vi "Get Vector - stdout.vi"(6 "no transpose\nfor reading":bool, 8 "error in (no error)":errorcluster, 9 "octave vector sizes":i32[](array[numeric]), 10 "variable name":string, 11 "GOLPI ref. in":T1={"pipe handle"={"lv_proc.dll file path"=path "", "process instance handle"=[]}, "fast read timeout [ms]"=500, "fast read settle time [ms]"=10, "fast read to multiple [ms]"=1, "max elements per input line"=100, "slow read timeout [ms]"=5000}) -> (0 "error out":errorcluster, 2 "vector":string[](array[string]), 3 "GOLPI ref. out":T1={"pipe handle"={"lv_proc.dll file path"=path "", "process instance handle"=[]}, "fast read timeout [ms]"=500, "fast read settle time [ms]"=10, "fast read to multiple [ms]"=1, "max elements per input line"=100, "slow read timeout [ms]"=5000}, 4 "value transposed?":bool)   [LabVIEW 2013, in "GOLPI library.lvlib"]
doc: "Reads vector variable from GNU Octave. Returns output as array of strings. Internaly converts row vector to column for simpler parsing of long vectors. It means complex vectors are conjugated and strings are incorrectly parsed. If 'no transpose for reading' is set true, function reads row vectors as rows."
uses:
  GOLPI library.lvlib
  Type Definitions/GOLPI reference Type Def.ctl
  LV Process.lvlibp/Pipe Handle.ctl
  Type Definitions/Custom Error Codes Enum Type Def.vi
  LV Process.lvlibp
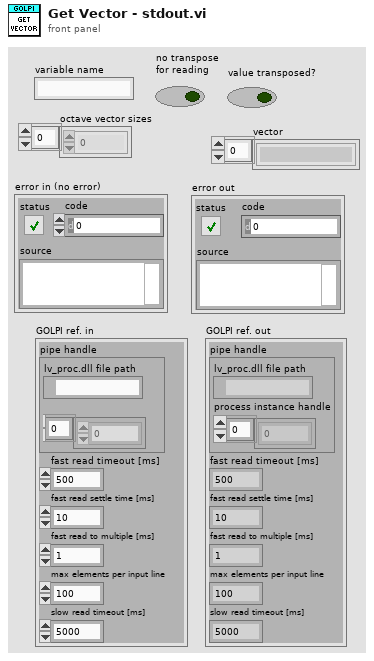
[diagram p1: front panel]
types:
  T1 = typedef "GOLPI library.lvlib/GOLPI reference Type Def.ctl" = cluster{"pipe handle":T2, "fast read timeout [ms]":u32, "fast read settle time [ms]":u32, "fast read to multiple [ms]":u32, "max elements per input line":u32, "slow read timeout [ms]":u32}
  T2 = typedef "LV Process.lvlibp/Pipe Handle.ctl" = cluster{"lv_proc.dll file path":path, "process instance handle":u32[]}
  T3 = typedef "GOLPI library.lvlib/Custom Error Codes Enum Type Def.vi" = enum16{"no error", "00 working directory PAR1 missing", "01 octave binary PAR1 missing", "02 octave report error PAR1", "03 empty output last cmd PAR1", "04 missing temporary file PAR1", "05 pwd PAR 1 not exist", "10 var PAR1 not string", "11 var PAR1 not num, scal, ~compl", "12 var PAR1 not num, scal, compl", "13 var PAR1 not num, vect, ~compl", "14 var PAR1 not num, vect, compl", "15 var PAR1 not num, mat, ~compl", "16 var PAR1 not num, mat, ~compl", "30 WARNING read timeout", "99 not finished"}
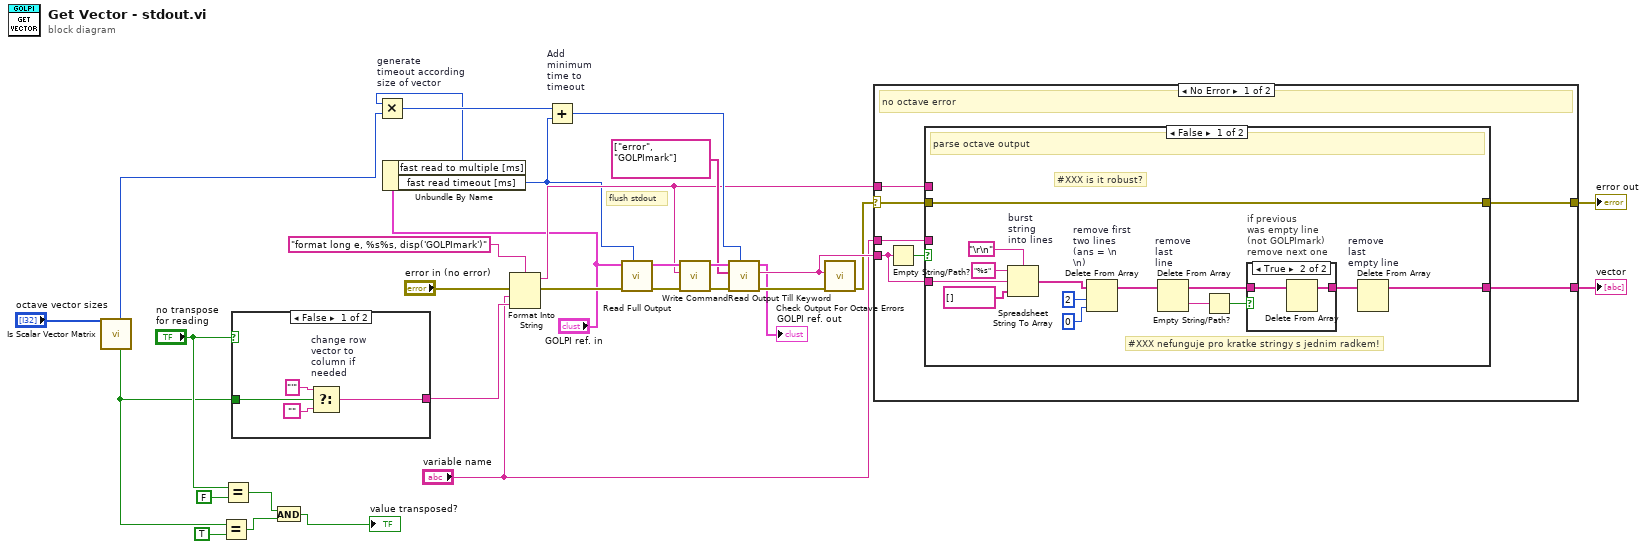
[diagram p0: block diagram]
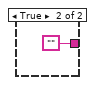
[diagram p2: hidden frame]
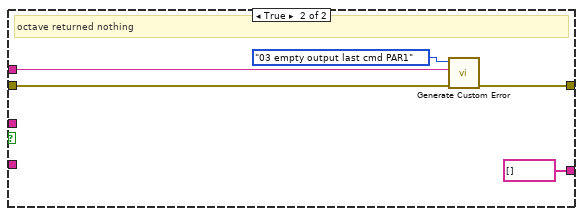
[diagram p4: hidden frame]
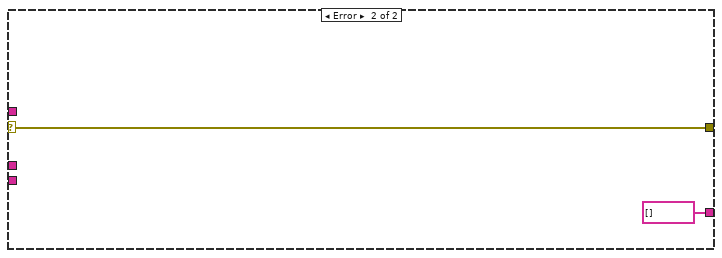
[diagram p5: hidden frame]
diagram:
  # "flush stdout"
  n1 = call "Is Scalar Vector Matrix.vi"("octave sizes"="octave vector sizes") -> ("row vector?"=w4:bool, "vector length"=w12:i32)  [unwired: 5 in, 4 out]
  n2 = Equal?(x=w4, y=TRUE) -> (x = y?=w2:bool)
  n3 = Equal?(x="no transpose\nfor reading", y=FALSE) -> (x = y?=w6:bool)
  n4 = case shown="False" "no transpose\nfor reading" {
    tunnel: [w33 ""] -> w28
    tunnel: w4 -> [w32 _]
    frame False {
      n5 = Select "change row\nvector to\ncolumn if\nneeded"(t="'", s=w32, f="") -> (s? t:f=w33:string)
    }
    frame True {
    }
  }
  n6 = And(x=w6, y=w2) -> (x .and. y?=→"value transposed?":bool)
  n7 = Unbundle By Name("GOLPI ref. in") -> ("fast read to multiple [ms]"=w8:u32, "fast read timeout [ms]"=w9:u32)
  n8 = Multiply "generate\ntimeout according\nsize of vector"(x=w8, y=w12) -> (x*y=w24:u32)
  n9 = Format Into String(format string="format long e, %s%s, disp('GOLPImark')", error in="error in (no error)", "variable name", w28) -> (resulting string=w14:string, error out=w20:errorcluster)  [unwired: 1 in]
  n10 = Add "Add\nminimum\ntime to\ntimeout"(x=w24, y=w9) -> (x+y=w23:u32)
  n11 = call "Read Full Output.vi"("timeout [ms]"=w9, "error in"=w20, "GOLPI ref. in"="GOLPI ref. in") -> ("error out"=w21:errorcluster, "GOLPI ref. out"=w22:T1)  [unwired: 5 in, 2 out]
  n12 = call "Write Command.vi"("error in"=w21, "command"=w14, "GOLPI ref. in"=w22) -> ("error out"=w25:errorcluster, "GOLPI ref. out"=w30:T1)  [unwired: 7 in]
  n13 = call "Read Output Till Keyword.vi"("timeout [ms]"=w23, "error in"=w25, "keywords"=string[] ["error", "GOLPImark"], "GOLPI ref. in"=w30) -> ("error out"=w31:errorcluster, "read buffer"=w19:string, "GOLPI ref. out"=→"GOLPI ref. out":T1)  [unwired: 4 in, 1 out]
  n14 = call "Check Output For Octave Errors.vi"("error in"=w31, "read buffer"=w19) -> ("error out"=w15:errorcluster)  [unwired: 9 in]
  n15 = case shown="No Error" w15 {
    selector: w15 -> [w40 w67]
    tunnel: w19 -> [w39 _]
    tunnel: "variable name" -> [w43 _]
    tunnel: [w42 string[] []] -> w17
    tunnel: [w41 w67] -> w16
    tunnel: w14 -> [w37 _]
    frame No Error {
      # "no octave error"
      n16 = Empty String/Path?(string/path=w39) -> (empty?=w38:bool)
      n17 = case shown="False" w38 {
        tunnel: w39 -> [w53 _]
        tunnel: w43 -> [_ _]
        tunnel: [w44 string[] []] -> w42
        tunnel: w40 -> [w57 w63]
        tunnel: [w57 w62] -> w41
        tunnel: w37 -> [_ w61]
        frame False {
          # "#XXX is it robust?"
          # "#XXX nefunguje pro kratke stringy s jednim radkem!"
          # "parse octave output"
          n18 = Spreadsheet String To Array "burst\nstring\ninto lines"(delimiter (Tab)="\r\n", format string="%s", spreadsheet string=w53, array type (2D Dbl)=string[] []) -> (array=w52:string[])
          n19 = Delete From Array "remove first\ntwo lines\n(ans = \\n\n\\n)"(array=w52, length=2, index=0) -> (array with subset deleted=w49:string[])  [unwired: 1 out]
          n20 = Delete From Array "remove\nlast\nline"(array=w49) -> (deleted portion=w48:string, array with subset deleted=w47:string[])  [unwired: 2 in]
          n21 = Empty String/Path?(string/path=w48) -> (empty?=w45:bool)
          n22 = case "if previous\nwas empty line\n(not GOLPImark)\nremove next one" shown="True" w45 {
            tunnel: w47 -> [w58 w60]
            tunnel: [w58 w59] -> w46
            frame False {
            }
            frame True {
              n23 = Delete From Array(array=w60) -> (array with subset deleted=w59:string[])  [unwired: 2 in, 1 out]
            }
          }
          n24 = Delete From Array "remove\nlast\nempty line"(array=w46) -> (array with subset deleted=w44:string[])  [unwired: 2 in, 1 out]
        }
        frame True {
          # "octave returned nothing"
          n25 = call "Generate Custom Error.vi"("error in"=w63, "PAR1"=w61, "GOLPI error"=Custom_Error_Codes_Enum_Type_Def.vi."03 empty output last cmd PAR1" ("Enum")) -> ("error out"=w62:errorcluster)  [unwired: 8 in]
        }
      }
    }
    frame Error {
    }
  }
  "error out" <- w16
  "vector" <- w17
